vi "createResponseParser.vi"(8 "error in (no error)":errorcluster, 11 "IOvenFactory in":refnum<class "IOvenFactory.lvclass">) -> (0 "error out":errorcluster, 2 "responseParser":refnum<class "IResponseParser.lvclass">, 3 "IOvenFactory out":refnum<class "IOvenFactory.lvclass">)   [LabVIEW 2023, in "AbstractFactory.lvlib" / "IOvenFactory.lvclass"]
uses:
  IOvenFactory.lvclass
  IResponseParser/IResponseParser.lvclass
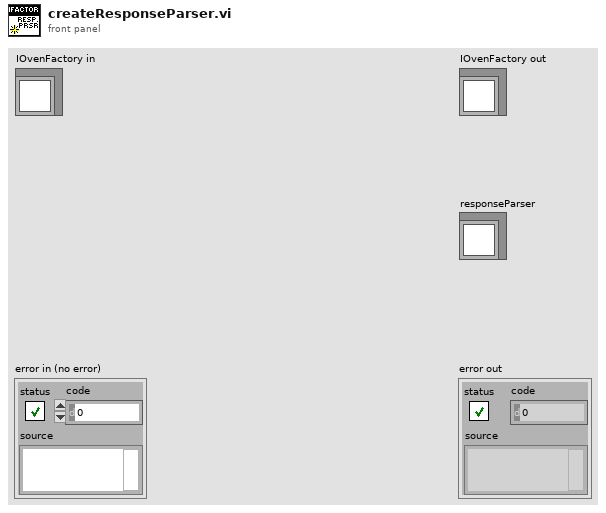
[diagram p1: front panel]
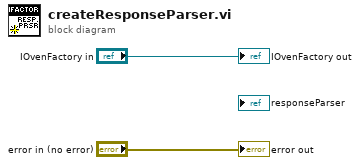
[diagram p0: block diagram]
diagram:
  "error out" <- "error in (no error)"
  "IOvenFactory out" <- "IOvenFactory in"
